vi "GetHSV.vi"(0 "ColorHLV in":refnum<class "ColorHSV.lvclass">, 11 "error in (no error)":errorcluster) -> (4 "ColorHLV out":refnum<class "ColorHSV.lvclass">, 6 "H (°)":dbl, 8 "S (%)":dbl, 10 "V (%)":dbl, 15 "error out":errorcluster)   [LabVIEW 2021, in "Picture2D.lvlib" / "ColorHSV.lvclass"]
uses:
  ColorHSV.lvclass
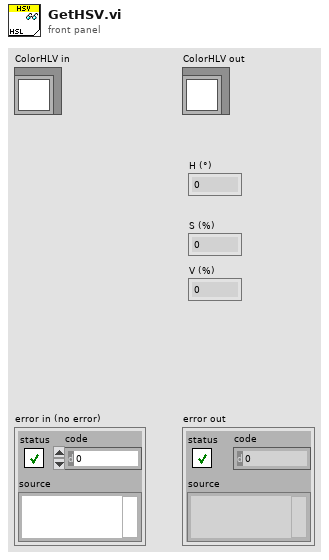
[diagram p1: front panel]
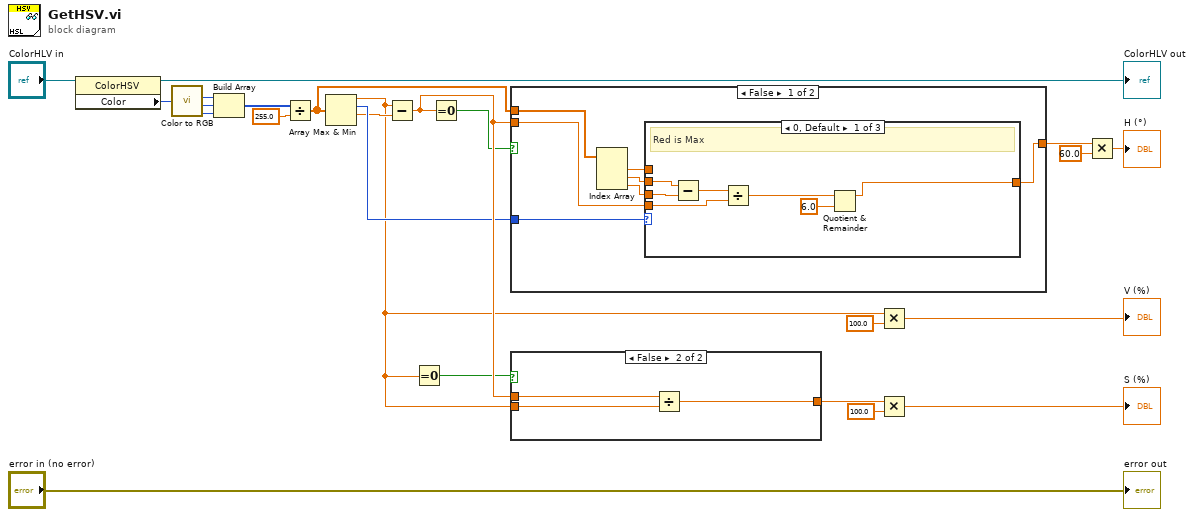
[diagram p0: block diagram]
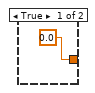
[diagram p2: hidden frame]
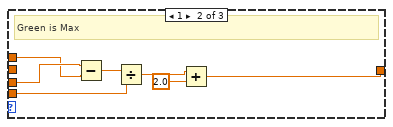
[diagram p3: hidden frame]
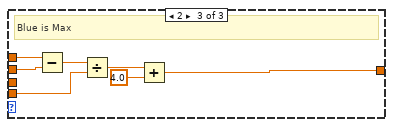
[diagram p4: hidden frame]
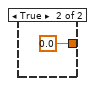
[diagram p5: hidden frame]
diagram:
  n1 = property class="ColorHSV"(reference="ColorHLV in") -> (reference out=→"ColorHLV out":refnum<class "ColorHSV.lvclass">, "Color"=w21:u32)  [unwired: 1 in, 1 out]
  n2 = call <vilib>:"Color to RGB.vi"("Color"=w21) -> ("R"=w12:u8, "G"=w11:u8, "B"=w10:u8)  [unwired: 1 out]
  n3 = Build Array(w12, w11, w10) -> (w20:u8[])
  n4 = Divide(x=w20, y=255.0 ("x")) -> (x/y=w18:dbl[])
  n5 = Array Max & Min(array=w18) -> (max value=w1:dbl, max index (indices)=w8:i32, min value=w7:dbl)  [unwired: 1 out]
  n6 = Subtract(x=w1, y=w7) -> (x-y=w9:dbl)
  n7 = Equal To 0?(x=w1) -> (x = 0?=w2:bool)
  n8 = Equal To 0?(x=w9) -> (x = 0?=w6:bool)
  n9 = case shown="False" w6 {
    tunnel: [w30 0.0] -> w17
    tunnel: w8 -> [w31 _]
    tunnel: w18 -> [w29 _]
    tunnel: w9 -> [w25 _]
    frame False {
      n10 = Index Array(array=w29) -> (element #1=w28:dbl, element #2=w27:dbl, element #3=w26:dbl)  [unwired: 3 in]
      n11 = case shown="0, Default" w31 {
        tunnel: w25 -> [w37 w43 w51]
        tunnel: [w32 w39 w49] -> w30
        tunnel: w28 -> [_ w44 w48]
        tunnel: w27 -> [w36 _ w47]
        tunnel: w26 -> [w35 w45 _]
        frame 0, Default {
          # "Red is Max"
          n12 = Subtract(x=w36, y=w35) -> (x-y=w38:dbl)
          n13 = Divide(x=w38, y=w37) -> (x/y=w34:dbl)
          n14 = Quotient & Remainder(x=w34, y=6.0) -> (x-y*floor(x/y)=w32:dbl)  [unwired: 1 out]
        }
        frame 1 {
          # "Green is Max"
          n15 = Subtract(x=w45, y=w44) -> (x-y=w42:dbl)
          n16 = Divide(x=w42, y=w43) -> (x/y=w41:dbl)
          n17 = Add(x=w41, y=2.0) -> (x+y=w39:dbl)
        }
        frame 2 {
          # "Blue is Max"
          n18 = Subtract(x=w48, y=w47) -> (x-y=w52:dbl)
          n19 = Divide(x=w52, y=w51) -> (x/y=w50:dbl)
          n20 = Add(x=w50, y=4.0) -> (x+y=w49:dbl)
        }
      }
    }
    frame True {
    }
  }
  n21 = case shown="False" w2 {
    tunnel: [0.0 ("y") w55] -> w13
    tunnel: w9 -> [_ w57]
    tunnel: w1 -> [_ w56]
    frame True {
    }
    frame False {
      n22 = Divide(x=w57, y=w56) -> (x/y=w55:dbl)
    }
  }
  n23 = Multiply(x=w1, y=100.0) -> (x*y=→"V (%)":dbl)
  n24 = Multiply(x=w13, y=100.0) -> (x*y=→"S (%)":dbl)
  n25 = Multiply(x=w17, y=60.0) -> (x*y=→"H (°)":dbl)
  "error out" <- "error in (no error)"
